vi "Fit Roll Axis(SubVI).vi"(8 "error in (no error)":errorcluster, 11 "Array of Joint Positions in":dbl[][](array[numeric])) -> (0 "error out":errorcluster, 3 "Roll":dbl)   [LabVIEW 2014]
uses:
  <vilib>/Analysis/NI_AALPro.lvlib
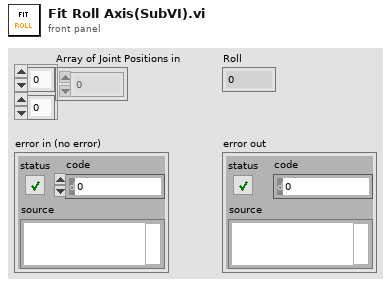
[diagram p1: front panel]
types:
  T1 = enum16{"hip centre", "spine", "shoulder centre", "head", "shoulder left", "elbow left", "wrist left", "hand left", "shoulder right", "elbow right", "wrist right", "hand right", "hip left", "knee left", "ankle left", "foot left", "hip right", "knee right", "ankle right", "foot right"}
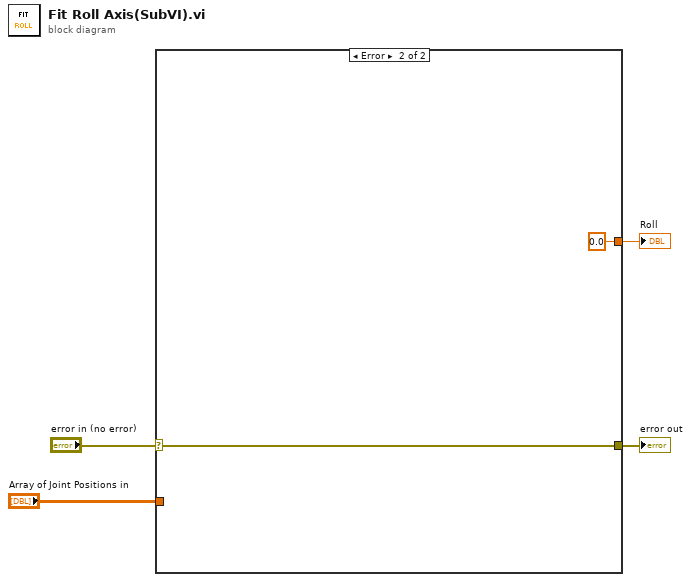
[diagram p0: block diagram]
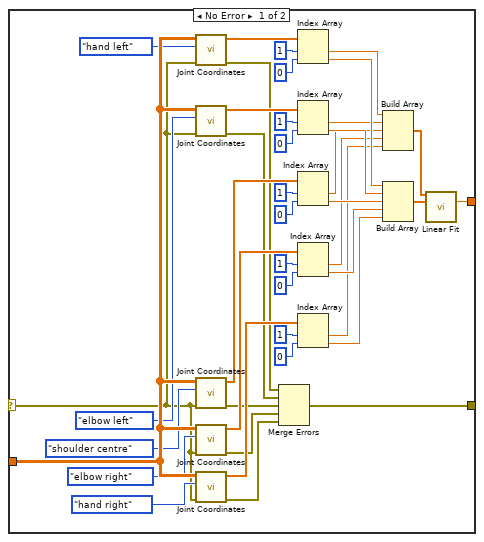
[diagram p2: hidden frame]
diagram:
  n1 = case shown="Error" "error in (no error)" {
    selector: "error in (no error)" -> [w5 w47]
    tunnel: "Array of Joint Positions in" -> [w35 _]
    tunnel: [w34 w47] -> w3
    tunnel: [w33 0.0 ("slope")] -> w2
    frame No Error {
      n2 = call <vilib>:"Joint Coordinates.vi"("error in (no error)"=w5, "Joint 1"=T1."hand left", "Array of Joint Positions"=w35) -> ("error out"=w11:errorcluster, "Joint Coordinates"=w21:dbl[])  [unwired: 7 in]
      n3 = call <vilib>:"Joint Coordinates.vi"("error in (no error)"=w5, "Joint 1"=T1."elbow left", "Array of Joint Positions"=w35) -> ("error out"=w12:errorcluster, "Joint Coordinates"=w22:dbl[])  [unwired: 7 in]
      n4 = call <vilib>:"Joint Coordinates.vi"("error in (no error)"=w5, "Joint 1"=T1."shoulder centre", "Array of Joint Positions"=w35) -> ("error out"=w13:errorcluster, "Joint Coordinates"=w23:dbl[])  [unwired: 7 in]
      n5 = call <vilib>:"Joint Coordinates.vi"("error in (no error)"=w5, "Joint 1"=T1."elbow right", "Array of Joint Positions"=w35) -> ("error out"=w14:errorcluster, "Joint Coordinates"=w25:dbl[])  [unwired: 7 in]
      n6 = call <vilib>:"Joint Coordinates.vi"("error in (no error)"=w5, "Joint 1"=T1."hand right", "Array of Joint Positions"=w35) -> ("error out"=w15:errorcluster, "Joint Coordinates"=w24:dbl[])  [unwired: 7 in]
      n7 = Merge Errors(w11, w12, w13, w14, w15) -> (w34:errorcluster)
      n8 = Index Array(array=w21, index #1=1 ("index"), index #2=0 ("index")) -> (element #1=w26:dbl, element #2=w37:dbl)
      n9 = Index Array(array=w22, index #1=1 ("index"), index #2=0 ("index")) -> (element #1=w27:dbl, element #2=w41:dbl)
      n10 = Index Array(array=w23, index #1=1 ("index"), index #2=0 ("index")) -> (element #1=w28:dbl, element #2=w43:dbl)
      n11 = Index Array(array=w25, index #1=1 ("index"), index #2=0 ("index")) -> (element #1=w29:dbl, element #2=w39:dbl)
      n12 = Index Array(array=w24, index #1=1 ("index"), index #2=0 ("index")) -> (element #1=w30:dbl, element #2=w45:dbl)
      n13 = Build Array(w26, w27, w28, w29, w30) -> (w32:dbl[])
      n14 = Build Array(w37, w41, w43, w39, w45) -> (w31:dbl[])
      n15 = call <vilib>:"Linear Fit.vi"("Y"=w32, "X"=w31) -> ("slope"=w33:dbl)  [unwired: 9 in, 4 out]
    }
    frame Error {
    }
  }
  "error out" <- w3
  "Roll" <- w2
